vi "Create Axis Object.vi"(7 "Actual Transform In":T1, 8 "error in (no error)":errorcluster, 10 "3D Plot.lvclass in":refnum<class "3D Plot.lvclass">, 11 "Axis Object In":refnum<vi>) -> (0 "error out":errorcluster, 2 "3D Plot.lvclass out":refnum<class "3D Plot.lvclass">, 3 "Axis Object Out":refnum<vi>, 5 "Actual Transform Out":T1)   [LabVIEW 2020, in "3D Plot.lvclass"]
uses:
  <vilib>/Math Plots/3D Math Plots/3D Plot/3D Plot/3D Plot.lvclass
  <vilib>/Math Plots/3D Math Plots/3D Plot/3D Plot/Typedef/Actual Transform.ctl
  <vilib>/Math Plots/3D Math Plots/3D Plot/3D Plot/Typedef/Range Clusters.ctl
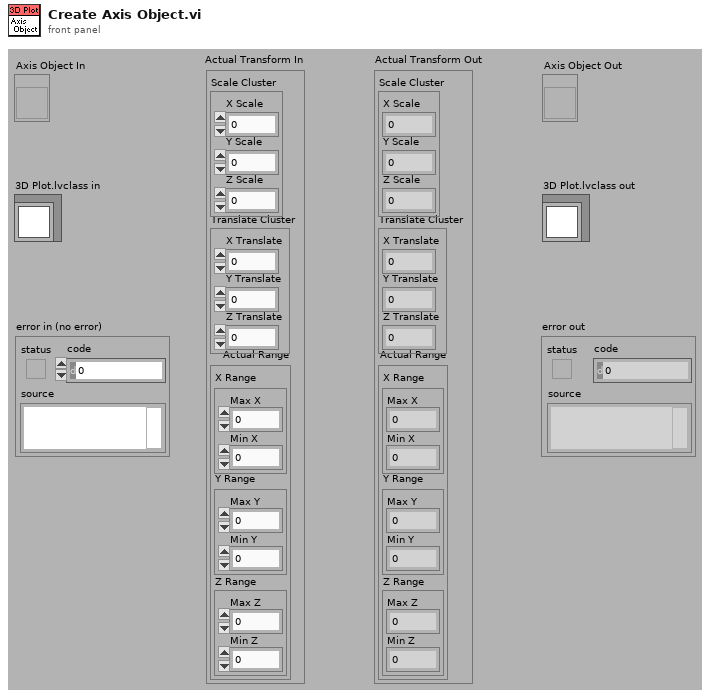
[diagram p1: front panel]
types:
  T1 = typedef "3D Plot.lvclass/Actual Transform.ctl" = cluster{"Scale Cluster":cluster{"X Scale":sgl, "Y Scale":sgl, "Z Scale":sgl}, "Translate Cluster":cluster{"X Translate":sgl, "Y Translate":sgl, "Z Translate":sgl}, "Actual Range":T2}
  T2 = typedef "3D Plot.lvclass/Range Clusters.ctl" = cluster{"X Range":cluster{"Max X":sgl, "Min X":sgl}, "Y Range":cluster{"Max Y":sgl, "Min Y":sgl}, "Z Range":cluster{"Max Z":sgl, "Min Z":sgl}}
  T3 = typedef "3D Plot.lvclass/Tick Array Cluster.ctl" = cluster{"X Tick Array":T4, "Y Tick Array":T4, "Z Tick Array":T4}
  T4 = typedef "3D Plot.lvclass/Tick Array.ctl" = cluster{"Label":bool, "Show Tick":bool, "Show Line":bool, "Value Numeric":sgl, "Value String":string}[]
  T5 = typedef "3D Plot.lvclass/Label Width.ctl" = cluster{"X Label Width":sgl, "Opposite X Label Width":sgl, "Y Label Width":sgl, "Opposite Y Label Width":sgl, "Z Label Width":sgl, "Opposite Z Label Width":sgl}
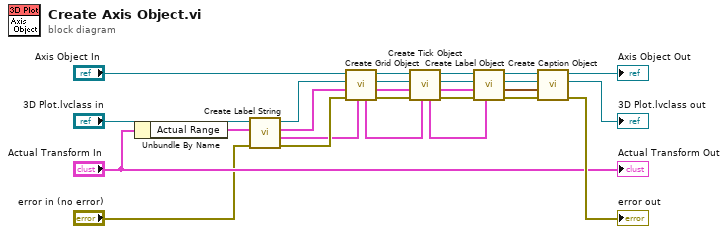
[diagram p0: block diagram]
diagram:
  n1 = Unbundle By Name("Actual Transform In") -> ("Actual Range"=w4:T2)
  n2 = call <vilib>:"Create Label String.vi"("error in (no error)"="error in (no error)", "Actual Range In"=w4, "3D Plot.lvclass in"="3D Plot.lvclass in") -> ("error out"=w20:errorcluster, "Label Cluster"=w2:T3, "Actual Range Out"=w3:T2, "3D Plot.lvclass out"=w7:refnum<class "3D Plot.lvclass">)  [unwired: 1 in, 4 out]
  n3 = call <vilib>:"Create Grid Object.vi"("Label Cluster In"=w2, "error in (no error)"=w20, "Actual Range In"=w3, "3D Plot.lvclass in"=w7, "Axis Object In"="Axis Object In") -> ("error out"=w21:errorcluster, "Actual Range Out"=w22:T2, "3D Plot.lvclass out"=w5:refnum<class "3D Plot.lvclass">, "Axis Object Out"=w26:refnum<vi>, "Label Cluster Out"=w23:T3)  [unwired: 1 in, 1 out]
  n4 = call <vilib>:"Create Tick Object.vi"("Label Cluster In"=w23, "error in (no error)"=w21, "Actual Range In"=w22, "3D Plot.lvclass in"=w5, "Axis Object In"=w26) -> ("error out"=w14:errorcluster, "Actual Range Out"=w15:T2, "3D Plot.lvclass out"=w17:refnum<class "3D Plot.lvclass">, "Axis Object Out"=w18:refnum<vi>, "Label Cluster Out"=w16:T3)  [unwired: 1 in, 1 out]
  n5 = call <vilib>:"Create Label Object.vi"("Label Cluster In"=w16, "error in (no error)"=w14, "Actual Range In"=w15, "3D Plot.lvclass in"=w17, "Axis Object In"=w18) -> ("error out"=w10:errorcluster, "Label Width"=w11:T5, "3D Plot.lvclass out"=w12:refnum<class "3D Plot.lvclass">, "Axis Object Out"=w13:refnum<vi>)  [unwired: 1 in, 2 out]
  n6 = call <vilib>:"Create Caption Object.vi"("error in (no error)"=w10, "Label Width"=w11, "3D Plot.lvclass in"=w12, "Axis Object In"=w13) -> ("error out"=→"error out":errorcluster, "3D Plot.lvclass out"=→"3D Plot.lvclass out":refnum<class "3D Plot.lvclass">, "Axis Object Out"=→"Axis Object Out":refnum<vi>)  [unwired: 5 out]
  "Actual Transform Out" <- "Actual Transform In"
